vi "BRig_RT__Case_Exp__State_initTrial__v2.vi"(0 "input_dataCurrent":u16[](array[numeric]), 9 "input_dataBlock":u16[][](array[numeric]), 11 "input_dataTrial":u16[][](array[numeric]), 12 "input_dataExp":u16[](array[numeric])) -> (1 "output_iTrial":u16, 2 "output_nTrial":u16, 3 "output_SolenoidReward":bool, 4 "output_dataCurrent":u16[](array[numeric]), 10 "output_dataBlock":u16[][](array[numeric]), 15 "output_dataTrial":u16[][](array[numeric]))   [LabVIEW 2014]
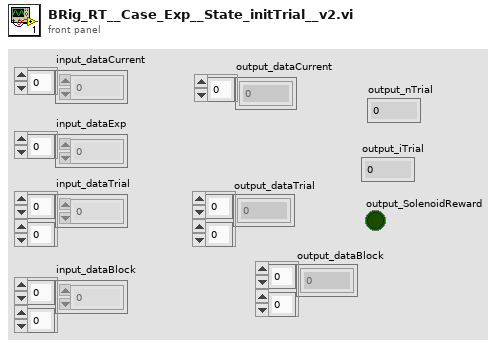
[diagram p1: front panel]
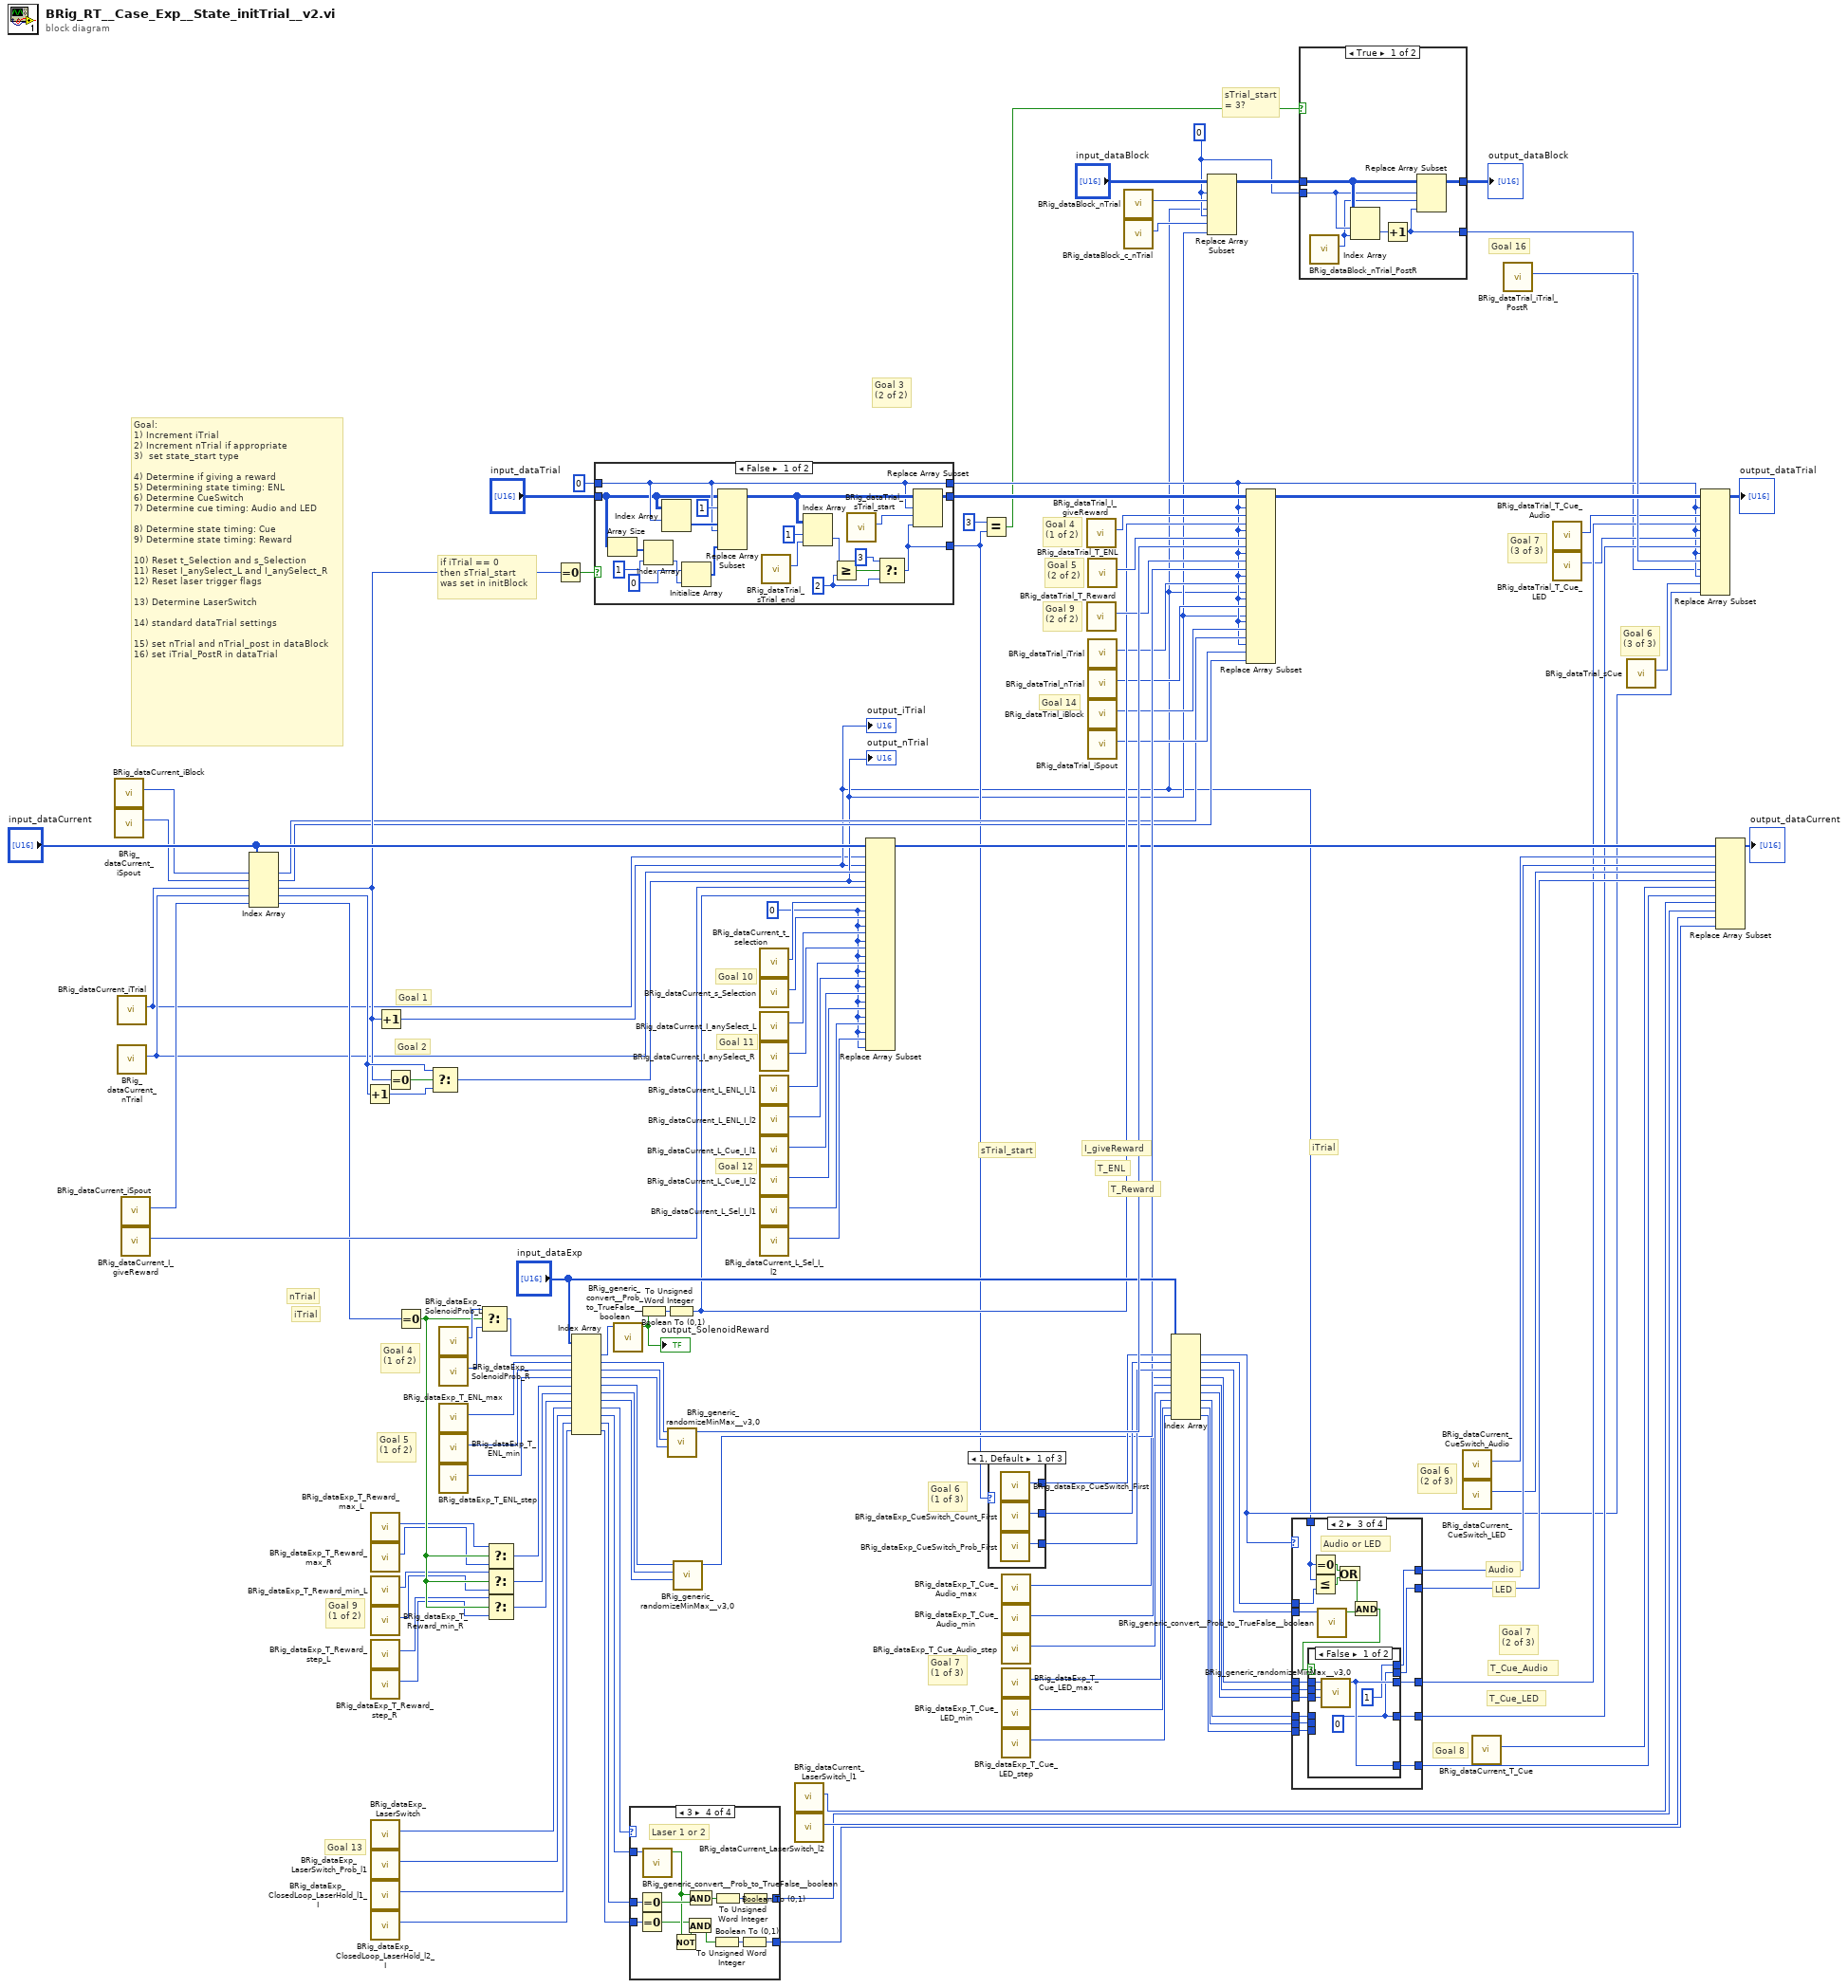
[diagram p0: block diagram]
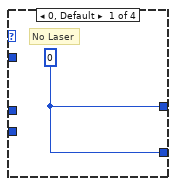
[diagram p3: hidden frame]
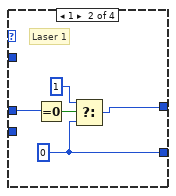
[diagram p4: hidden frame]
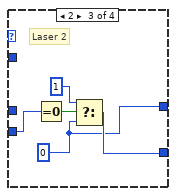
[diagram p5: hidden frame]
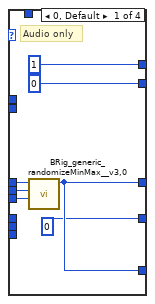
[diagram p6: hidden frame]
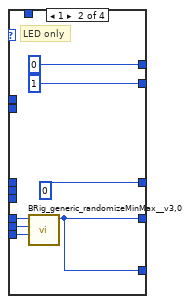
[diagram p7: hidden frame]
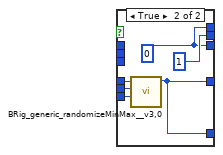
[diagram p8: hidden frame]
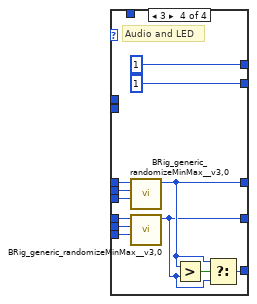
[diagram p9: hidden frame]
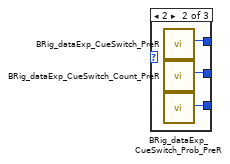
[diagram p10: hidden frame]
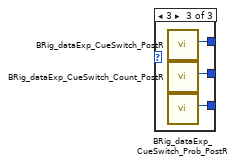
[diagram p11: hidden frame]
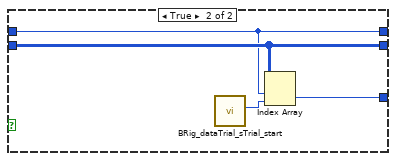
[diagram p12: hidden frame]
diagram:
  w6 = 0 ("disabled index (row)")
  w83 = u16 0 ("new element/subarray")
  # "Goal 16"
  # "Goal 6\n(3 of 3)"
  # "iTrial"
  # "sTrial_start\n= 3?"
  # "nTrial"
  # "Goal 14"
  # "Goal 13"
  # "iTrial"
  # "Goal 8"
  # "Goal 7\n(3 of 3)"
  # "Goal 7\n(2 of 3)"
  # "Goal 7\n(1 of 3)"
  # "T_Cue_LED"
  # "T_Cue_Audio"
  # "I_giveReward"
  # "Goal 4\n(1 of 2)"
  # "T_Reward"
  # "Goal 9\n(2 of 2)"
  # "Goal 9\n(1 of 2)"
  # "Goal 12"
  # "Goal 11"
  # "Goal 10"
  # "T_ENL"
  # "sTrial_start"
  # "LED"
  # "Audio"
  # "Goal 6\n(2 of 3)"
  # "Goal 6\n(1 of 3)"
  # "Goal 3\n(2 of 2)"
  # "Goal 5\n(2 of 2)"
  # "Goal 5\n(1 of 2)"
  # "Goal 4\n(1 of 2)"
  # "if iTrial == 0\nthen sTrial_start\nwas set in initBlock"
  # "Goal 2"
  # "Goal 1"
  # "Goal:\n1) Increment iTrial\n2) Increment nTrial if appropriate\n3)  set state_start type\n\n4) Determine if giving a reward\n5) Determining state timing: ENL\n6) Determine CueSwitch\n7) Determine cue timing: Audio and LED\n\n8) Determine state timing: Cue\n9) Determine state timing: Reward\n\n10) Reset t_Selection and s_Selection\n11) Reset I_anySelect_L and I_anySelect_R\n12) Reset laser trigger flags\n\n13) Determine LaserSwitch\n\n14) standard dataTrial settings\n\n15) set nTrial and nTrial_post in dataBlock\n16) set iTrial_PostR in dataTrial"
  n1 = call "BRig_dataCurrent_iBlock.vi"() -> ("output_iBlock"=w25:i32)  [unwired: 11 in]
  n2 = call "BRig_dataCurrent_iSpout.vi"() -> ("output_iSpout"=w24:i32)  [unwired: 11 in]
  n3 = call "BRig_dataCurrent_iTrial.vi"() -> ("output_iTrial"=w1:i32)  [unwired: 11 in]
  n4 = call "BRig_dataCurrent_nTrial.vi"() -> ("output_nTrial"=w4:i32)  [unwired: 11 in]
  n5 = call "BRig_dataCurrent_iSpout.vi"() -> ("output_iSpout"=w15:i32)  [unwired: 11 in]
  n6 = call "BRig_dataCurrent_I_giveReward.vi"() -> ("output_I_giveReward"=w117:i32)  [unwired: 11 in]
  n7 = Index Array(array="input_dataCurrent", index #1=w25, index #2=w24, index #3=w1, index #4=w4, index #5=w15) -> (element #1=w35:u16, element #2=w34:u16, element #3=w48:u16, element #4=w123:u16, element #5=w14:u16)
  n8 = Increment(x=w123) -> (x+1=w122:u16)
  n9 = call "BRig_dataExp_T_Reward_max_L.vi"() -> ("output_T_Reward_max_L"=w81:i32)  [unwired: 11 in]
  n10 = call "BRig_dataExp_T_Reward_max_R.vi"() -> ("output_T_Reward_max_R"=w80:i32)  [unwired: 11 in]
  n11 = call "BRig_dataExp_T_Reward_min_L.vi"() -> ("output_Tcycle_Reward_min_L"=w79:i32)  [unwired: 11 in]
  n12 = call "BRig_dataExp_T_Reward_min_R.vi"() -> ("output_T_Reward_min_R"=w78:i32)  [unwired: 11 in]
  n13 = call "BRig_dataExp_T_Reward_step_L.vi"() -> ("output_T_Reward_step_L"=w77:i32)  [unwired: 11 in]
  n14 = call "BRig_dataExp_T_Reward_step_R.vi"() -> ("output_T_Reward_step_R"=w76:i32)  [unwired: 11 in]
  n15 = call "BRig_dataExp_LaserSwitch.vi"() -> ("output_LaserSwitch"=w47:i32)  [unwired: 11 in]
  n16 = call "BRig_dataExp_LaserSwitch_Prob_l1.vi"() -> ("output_LaserSwitch_Probability_L1"=w46:i32)  [unwired: 11 in]
  n17 = call "BRig_dataExp_ClosedLoop_LaserHold_l1_I.vi"() -> ("output_CloseLoop_LaserHold_l1_I"=w20:i32)  [unwired: 11 in]
  n18 = call "BRig_dataExp_ClosedLoop_LaserHold_l2_I.vi"() -> ("output_CloseLoop_LaserHold_l2_I"=w19:i32)  [unwired: 11 in]
  n19 = Increment(x=w48) -> (x+1=w2:u16)
  "output_iTrial" <- w2
  n20 = Equal To 0?(x=w48) -> (x = 0?=w121:bool)
  n21 = Equal To 0?(x=w14) -> (x = 0?=w82:bool)
  n22 = Select(t=w123, s=w121, f=w122) -> (s? t:f=w3:u16)
  "output_nTrial" <- w3
  n23 = call "BRig_dataExp_SolenoidProb_L.vi"() -> ("output_SolenoidProbability_L"=w116:i32)  [unwired: 11 in]
  n24 = call "BRig_dataExp_SolenoidProb_R.vi"() -> ("output_SolenoidProbability_R"=w115:i32)  [unwired: 11 in]
  n25 = call "BRig_dataExp_T_ENL_max.vi"() -> ("output_T_ENL_max"=w109:i32)  [unwired: 11 in]
  n26 = call "BRig_dataExp_T_ENL_min.vi"() -> ("output_T_ENL_min"=w110:i32)  [unwired: 11 in]
  n27 = call "BRig_dataExp_T_ENL_step.vi"() -> ("output_T_ENL_step"=w111:i32)  [unwired: 11 in]
  n28 = Select(t=w116, s=w82, f=w115) -> (s? t:f=w114:i32)
  n29 = Select(t=w81, s=w82, f=w80) -> (s? t:f=w75:i32)
  n30 = Select(t=w79, s=w82, f=w78) -> (s? t:f=w74:i32)
  n31 = Select(t=w77, s=w82, f=w76) -> (s? t:f=w73:i32)
  n32 = Equal To 0?(x=w48) -> (x = 0?=w120:bool)
  n33 = Index Array(array="input_dataExp", index #1=w114, index #2=w109, index #3=w110, index #4=w111, index #5=w75, index #6=w74, index #7=w73, index #8=w47, index #9=w46, index #10=w20, index #11=w19) -> (element #1=w113:u16, element #2=w108:u16, element #3=w107:u16, element #4=w106:u16, element #5=w72:u16, element #6=w71:u16, element #7=w70:u16, element #8=w45:u16, element #9=w44:u16, element #10=w18:u16, element #11=w17:u16)
  n34 = case shown="False" w120 {
    tunnel: "input_dataTrial" -> [w130 w147]
    tunnel: [w141 w147] -> w105
    tunnel: 0 -> [w131 w146]
    tunnel: [w131 w146] -> w23
    tunnel: [w137 w144] -> w12
    frame False {
      w138 = u16 2 ("y")
      n35 = Array Size(array=w130) -> (size(s)=w129:i32[])
      n36 = Index Array(array=w129, index=1) -> (element=w127:i32)
      n37 = Index Array(array=w130, index (row)=w131) -> (element=w134:u16[])  [unwired: 1 in]
      n38 = Initialize Array(u16 0 ("index"), w127) -> (w125:u16[])
      n39 = Replace Array Subset(array=w130, new element #1=w134, index (row) #1=1 ("index (row)"), new element #2=w125, index (row) #2=w131) -> (w132:u16[][])  [unwired: 2 in]
      n40 = call "BRig_dataTrial_sTrial_end.vi"() -> ("output_sTrial_end"=w143:i32)  [unwired: 11 in]
      n41 = Index Array(array=w132, index (row)=1 ("disabled index (row)"), index (col)=w143) -> (element=w142:u16)
      n42 = Greater Or Equal?(x=w142, y=w138) -> (x >= y?=w140:bool)
      n43 = call "BRig_dataTrial_sTrial_start.vi"() -> ("output_sTrial_start"=w136:i32)  [unwired: 11 in]
      n44 = Select(t=u16 3 ("y"), s=w140, f=w138) -> (s? t:f=w137:u16)
      n45 = Replace Array Subset(array=w132, new element=w137, index (row)=w131, index (col)=w136) -> (w141:u16[][])
    }
    frame True {
      n46 = call "BRig_dataTrial_sTrial_start.vi"() -> ("output_sTrial_start"=w145:i32)  [unwired: 11 in]
      n47 = Index Array(array=w147, index (row)=w146, index (col)=w145) -> (element=w144:u16)
    }
  }
  n48 = call "BRig_generic_convert__Prob_to_TrueFalse__boolean.vi"("input_probability_u16"=w113) -> ("output_TF"=w112:bool)  [unwired: 10 in]
  "output_SolenoidReward" <- w112
  n49 = case shown="3" w45 {
    tunnel: [w148 w149 w154 w168] -> w42
    tunnel: [w148 w150 w155 w167] -> w41
    tunnel: w44 -> [_ _ _ w171]
    tunnel: w18 -> [_ w153 _ w166]
    tunnel: w17 -> [_ _ w156 w165]
    frame 0, Default {
      w148 = u16 0
      # "No Laser"
    }
    frame 1 {
      w150 = u16 0
      # "Laser 1"
      n50 = Equal To 0?(x=w153) -> (x = 0?=w152:bool)
      n51 = Select(t=u16 1, s=w152, f=w150) -> (s? t:f=w149:u16)
    }
    frame 2 {
      w154 = u16 0
      # "Laser 2"
      n52 = Equal To 0?(x=w156) -> (x = 0?=w158:bool)
      n53 = Select(t=u16 1, s=w158, f=w154) -> (s? t:f=w155:u16)
    }
    frame 3 {
      # "Laser 1 or 2"
      n54 = Equal To 0?(x=w166) -> (x = 0?=w164:bool)
      n55 = Equal To 0?(x=w165) -> (x = 0?=w160:bool)
      n56 = call "BRig_generic_convert__Prob_to_TrueFalse__boolean.vi"("input_probability_u16"=w171) -> ("output_TF"=w163:bool)  [unwired: 10 in]
      n57 = Not(x=w163) -> (.not. x?=w161:bool)
      n58 = And(x=w160, y=w161) -> (x .and. y?=w159:bool)
      n59 = And(x=w163, y=w164) -> (x .and. y?=w162:bool)
      n60 = Boolean To (0,1)(Boolean=w159) -> (0, 1=w170:i16)
      n61 = Boolean To (0,1)(Boolean=w162) -> (0, 1=w169:i16)
      n62 = To Unsigned Word Integer(number=w170) -> (unsigned 16bit integer=w167:u16)
      n63 = To Unsigned Word Integer(number=w169) -> (unsigned 16bit integer=w168:u16)
    }
  }
  n64 = Boolean To (0,1)(Boolean=w112) -> (0, 1=w124:i16)
  n65 = To Unsigned Word Integer(number=w124) -> (unsigned 16bit integer=w66:u16)
  n66 = call "BRig_generic_randomizeMinMax__v3,0.vi"("Input_Increment"=w106, "Input_Min"=w107, "Input_Max"=w108) -> ("Output"=w103:u16)  [unwired: 8 in]
  n67 = call "BRig_generic_randomizeMinMax__v3,0.vi"("Input_Increment"=w70, "Input_Min"=w71, "Input_Max"=w72) -> ("Output"=w68:u16)  [unwired: 8 in]
  n68 = call "BRig_dataCurrent_t_selection.vi"() -> ("output_t_selection"=w93:i32)  [unwired: 11 in]
  n69 = call "BRig_dataCurrent_s_Selection.vi"() -> ("output_s_Selection"=w92:i32)  [unwired: 11 in]
  n70 = call "BRig_dataCurrent_I_anySelect_L.vi"() -> ("output_IanySelect_L"=w91:i32)  [unwired: 11 in]
  n71 = call "BRig_dataCurrent_I_anySelect_R.vi"() -> ("output_IanySelect_R"=w90:i32)  [unwired: 11 in]
  n72 = call "BRig_dataCurrent_L_ENL_I_l1.vi"() -> ("output_L_ENL_I_l1"=w89:i32)  [unwired: 11 in]
  n73 = call "BRig_dataCurrent_L_ENL_I_l2.vi"() -> ("output_L_ENL_I_l2"=w88:i32)  [unwired: 11 in]
  n74 = call "BRig_dataCurrent_L_Cue_I_l1.vi"() -> ("output_L_Cue_I_l1"=w87:i32)  [unwired: 11 in]
  n75 = call "BRig_dataCurrent_L_Cue_I_l2.vi"() -> ("output_L_Cue_I_l2"=w86:i32)  [unwired: 11 in]
  n76 = call "BRig_dataCurrent_L_Sel_I_l1.vi"() -> ("output_L_Sel_I_l1"=w85:i32)  [unwired: 11 in]
  n77 = call "BRig_dataCurrent_L_Sel_I_l2.vi"() -> ("output_L_Sel_I_l2"=w84:i32)  [unwired: 11 in]
  n78 = call "BRig_dataCurrent_LaserSwitch_l1.vi"() -> ("output_LaserSwitch_l1"=w40:i32)  [unwired: 11 in]
  n79 = call "BRig_dataCurrent_LaserSwitch_l2.vi"() -> ("output_LaserSwitch_l2"=w43:i32)  [unwired: 11 in]
  n80 = Replace Array Subset(array="input_dataCurrent", new element #1=w2, index #1=w1, new element #2=w3, index #2=w4, new element #3=w66, index #3=w117, new element #4=w83, index #4=w93, new element #5=w83, index #5=w92, new element #6=w83, index #6=w91, new element #7=w83, index #7=w90, new element #8=w83, index #8=w89, new element #9=w83, index #9=w88, new element #10=w83, index #10=w87, new element #11=w83, index #11=w86, new element #12=w83, index #12=w85, new element #13=w83, index #13=w84) -> (w32:u16[])
  n81 = Equal?(x=u16 3 ("y"), y=w12) -> (x = y?=w7:bool)
  n82 = case shown="1, Default" w12 {
    tunnel: [w174 w175 w180] -> w100
    tunnel: [w173 w176 w179] -> w99
    tunnel: [w172 w177 w178] -> w98
    frame 1, Default {
      n83 = call "BRig_dataExp_CueSwitch_First.vi"() -> ("output_CueSwitch_First"=w174:i32)  [unwired: 11 in]
      n84 = call "BRig_dataExp_CueSwitch_Count_First.vi"() -> ("output_CueSwitch_Count_First"=w173:i32)  [unwired: 11 in]
      n85 = call "BRig_dataExp_CueSwitch_Prob_First.vi"() -> ("output_CueSwitch_Prob_First"=w172:i32)  [unwired: 11 in]
    }
    frame 2 {
      n86 = call "BRig_dataExp_CueSwitch_PreR.vi"() -> ("output_CueSwitch_PreR"=w175:i32)  [unwired: 11 in]
      n87 = call "BRig_dataExp_CueSwitch_Count_PreR.vi"() -> ("output_CueSwitch_Count_PreR"=w176:i32)  [unwired: 11 in]
      n88 = call "BRig_dataExp_CueSwitch_Prob_PreR.vi"() -> ("output_CueSwitch_Prob_PreR"=w177:i32)  [unwired: 11 in]
    }
    frame 3 {
      n89 = call "BRig_dataExp_CueSwitch_PostR.vi"() -> ("output_CueSwitch_PostR"=w180:i32)  [unwired: 11 in]
      n90 = call "BRig_dataExp_CueSwitch_Count_PostR.vi"() -> ("output_CueSwitch_Count_PostR"=w179:i32)  [unwired: 11 in]
      n91 = call "BRig_dataExp_CueSwitch_Prob_PostR.vi"() -> ("output_CueSwitch_Prob_PostR"=w178:i32)  [unwired: 11 in]
    }
  }
  n92 = call "BRig_dataExp_T_Cue_Audio_max.vi"() -> ("output_T_Cue_Audio_max"=w65:i32)  [unwired: 11 in]
  n93 = call "BRig_dataExp_T_Cue_Audio_min.vi"() -> ("output_T_Cue_Audio_min"=w64:i32)  [unwired: 11 in]
  n94 = call "BRig_dataExp_T_Cue_Audio_step.vi"() -> ("output_T_Cue_Audio_step"=w63:i32)  [unwired: 11 in]
  n95 = call "BRig_dataExp_T_Cue_LED_max.vi"() -> ("output_T_Cue_LED_max"=w62:i32)  [unwired: 11 in]
  n96 = call "BRig_dataExp_T_Cue_LED_min.vi"() -> ("output_T_Cue_LED_min"=w61:i32)  [unwired: 11 in]
  n97 = call "BRig_dataExp_T_Cue_LED_step.vi"() -> ("output_T_Cue_LED_step"=w60:i32)  [unwired: 11 in]
  n98 = call "BRig_dataTrial_I_giveReward.vi"() -> ("output_I_giveReward"=w67:i32)  [unwired: 11 in]
  n99 = call "BRig_dataTrial_T_Reward.vi"() -> ("output_T_Reward"=w69:i32)  [unwired: 11 in]
  n100 = call "BRig_dataTrial_T_ENL.vi"() -> ("output_T_ENL"=w104:i32)  [unwired: 11 in]
  n101 = call "BRig_dataTrial_iTrial.vi"() -> ("output_iTrial"=w39:i32)  [unwired: 11 in]
  n102 = call "BRig_dataTrial_nTrial.vi"() -> ("output_nTrial"=w38:i32)  [unwired: 11 in]
  n103 = call "BRig_dataTrial_iBlock.vi"() -> ("output_iBlock"=w37:i32)  [unwired: 11 in]
  n104 = call "BRig_dataTrial_iSpout.vi"() -> ("output_iSpout"=w36:i32)  [unwired: 11 in]
  n105 = call "BRig_dataBlock_nTrial.vi"() -> ("output_nTrial"=w9:i32)  [unwired: 11 in]
  n106 = call "BRig_dataBlock_c_nTrial.vi"() -> ("output_c_nTrial"=w8:i32)  [unwired: 11 in]
  n107 = Index Array(array="input_dataExp", index #1=w100, index #2=w99, index #3=w98, index #4=w65, index #5=w64, index #6=w63, index #7=w62, index #8=w61, index #9=w60) -> (element #1=w21:u16, element #2=w59:u16, element #3=w58:u16, element #4=w57:u16, element #5=w56:u16, element #6=w55:u16, element #7=w54:u16, element #8=w53:u16, element #9=w52:u16)
  n108 = Replace Array Subset(array="input_dataBlock", new element #1=w2, index (row) #1=w6, index (col) #1=w9, new element #2=w3, index (row) #2=w6, index (col) #2=w8) -> (w10:u16[][])
  n109 = Replace Array Subset(array=w105, new element #1=w66, index (row) #1=w23, index (col) #1=w67, new element #2=w103, index (row) #2=w23, index (col) #2=w104, new element #3=w68, index (row) #3=w23, index (col) #3=w69, new element #4=w2, index (row) #4=w23, index (col) #4=w39, new element #5=w3, index (row) #5=w23, index (col) #5=w38, new element #6=w35, index (row) #6=w23, index (col) #6=w37, new element #7=w34, index (row) #7=w23, index (col) #7=w36) -> (w31:u16[][])
  n110 = case shown="2" w21 {
    tunnel: [u16 1 u16 0 w199 u16 1] -> w96
    tunnel: [u16 0 u16 1 w198 u16 1] -> w94
    tunnel: w59 -> [_ _ w212 _]
    tunnel: w58 -> [_ _ w209 _]
    tunnel: w57 -> [w185 _ w205 w235]
    tunnel: w56 -> [w184 _ w204 w234]
    tunnel: w55 -> [w183 _ w203 w233]
    tunnel: w54 -> [_ w192 w197 w232]
    tunnel: w53 -> [_ w191 w196 w231]
    tunnel: w52 -> [_ w190 w195 w230]
    tunnel: [w182 u16 0 ("Output") w202 w228] -> w29
    tunnel: [u16 0 ("Output") w189 w200 w227] -> w28
    tunnel: [w182 w189 w201 w226] -> w49
    tunnel: w2 -> [_ _ w213 _]
    frame 0, Default {
      # "Audio only"
      n111 = call "BRig_generic_randomizeMinMax__v3,0.vi"("Input_Increment"=w183, "Input_Min"=w184, "Input_Max"=w185) -> ("Output"=w182:u16)  [unwired: 8 in]
    }
    frame 1 {
      # "LED only"
      n112 = call "BRig_generic_randomizeMinMax__v3,0.vi"("Input_Increment"=w190, "Input_Min"=w191, "Input_Max"=w192) -> ("Output"=w189:u16)  [unwired: 8 in]
    }
    frame 2 {
      # "Audio or LED"
      n113 = Equal To 0?(x=w213) -> (x = 0?=w211:bool)
      n114 = Less Or Equal?(x=w213, y=w212) -> (x <= y?=w210:bool)
      n115 = call "BRig_generic_convert__Prob_to_TrueFalse__boolean.vi"("input_probability_u16"=w209) -> ("output_TF"=w208:bool)  [unwired: 10 in]
      n116 = Or(x=w211, y=w210) -> (x .or. y?=w207:bool)
      n117 = And(x=w207, y=w208) -> (x .and. y?=w206:bool)
      n118 = case shown="False" w206 {
        tunnel: w205 -> [w219 _]
        tunnel: w204 -> [w218 _]
        tunnel: w203 -> [w217 _]
        tunnel: [w216 w220] -> w202
        tunnel: [w216 w222] -> w201
        tunnel: [w214 w222] -> w200
        tunnel: [u16 1 w220] -> w199
        tunnel: [w214 u16 1] -> w198
        tunnel: w197 -> [_ w225]
        tunnel: w196 -> [_ w224]
        tunnel: w195 -> [_ w223]
        frame False {
          w214 = u16 0
          n119 = call "BRig_generic_randomizeMinMax__v3,0.vi"("Input_Increment"=w217, "Input_Min"=w218, "Input_Max"=w219) -> ("Output"=w216:u16)  [unwired: 8 in]
        }
        frame True {
          w220 = u16 0
          n120 = call "BRig_generic_randomizeMinMax__v3,0.vi"("Input_Increment"=w223, "Input_Min"=w224, "Input_Max"=w225) -> ("Output"=w222:u16)  [unwired: 8 in]
        }
      }
    }
    frame 3 {
      # "Audio and LED"
      n121 = call "BRig_generic_randomizeMinMax__v3,0.vi"("Input_Increment"=w233, "Input_Min"=w234, "Input_Max"=w235) -> ("Output"=w228:u16)  [unwired: 8 in]
      n122 = call "BRig_generic_randomizeMinMax__v3,0.vi"("Input_Increment"=w230, "Input_Min"=w231, "Input_Max"=w232) -> ("Output"=w227:u16)  [unwired: 8 in]
      n123 = Greater?(x=w228, y=w227) -> (0:w229:bool)
      n124 = Select(t=w228, s=w229, f=w227) -> (s? t:f=w226:u16)
    }
  }
  n125 = case shown="True" w7 {
    tunnel: w10 -> [w243 w244]
    tunnel: [w241 w244] -> w33
    tunnel: [w238 _] -> w5
    tunnel: w6 -> [w240 _]
    frame True {
      n126 = call "BRig_dataBlock_nTrial_PostR.vi"() -> ("output_nTrial_PostR"=w239:i32)  [unwired: 11 in]
      n127 = Index Array(array=w243, index (row)=w240, index (col)=w239) -> (element=w242:u16)
      n128 = Increment(x=w242) -> (x+1=w238:u16)
      n129 = Replace Array Subset(array=w243, new element=w238, index (row)=w240, index (col)=w239) -> (w241:u16[][])
    }
    frame False {
    }
  }
  "output_dataBlock" <- w33
  n130 = call "BRig_dataCurrent_CueSwitch_Audio.vi"() -> ("output_CueSwitch_Audio"=w97:i32)  [unwired: 11 in]
  n131 = call "BRig_dataCurrent_CueSwitch_LED.vi"() -> ("output_CueSwitch_LED"=w95:i32)  [unwired: 11 in]
  n132 = call "BRig_dataCurrent_T_Cue.vi"() -> ("output_T_Cue"=w50:i32)  [unwired: 11 in]
  n133 = call "BRig_dataTrial_iTrial_PostR.vi"() -> ("output_iTrial_PostR"=w30:i32)  [unwired: 11 in]
  n134 = call "BRig_dataTrial_T_Cue_Audio.vi"() -> ("output_T_Cue_Audio"=w27:i32)  [unwired: 11 in]
  n135 = call "BRig_dataTrial_T_Cue_LED.vi"() -> ("output_T_Cue_LED"=w26:i32)  [unwired: 11 in]
  n136 = call "BRig_dataTrial_sCue.vi"() -> ("output_sCue"=w22:i32)  [unwired: 11 in]
  n137 = Replace Array Subset(array=w31, new element #1=w29, index (row) #1=w23, index (col) #1=w27, new element #2=w28, index (row) #2=w23, index (col) #2=w26, new element #3=w5, index (row) #3=w23, index (col) #3=w30, new element #4=w21, index (row) #4=w23, index (col) #4=w22) -> (→"output_dataTrial":u16[][])
  n138 = Replace Array Subset(array=w32, new element #1=w96, index #1=w97, new element #2=w94, index #2=w95, new element #3=w49, index #3=w50, new element #4=w42, index #4=w40, new element #5=w41, index #5=w43) -> (→"output_dataCurrent":u16[])
